vi "Get Revolutions.vi"(8 "error in (no error)":errorcluster, 11 "DriveMotors in":refnum<class "DriveMotors.lvclass">) -> (0 "error out":errorcluster, 2 "Revolutions":dbl, 3 "DriveMotors out":refnum<class "DriveMotors.lvclass">)   [LabVIEW 2013, in "DriveMotors.lvclass"]
uses:
  DriveMotors.lvclass
  DriveMotors.lvclass/DriveMotors.ctl
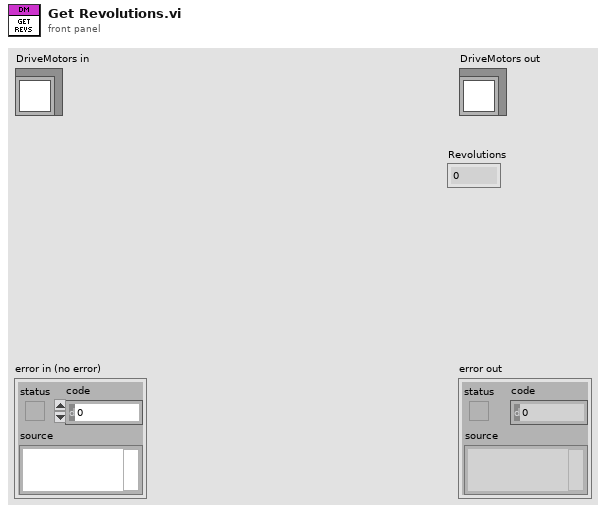
[diagram p1: front panel]
types:
  T1 = typedef "WPI_EncoderDevRef.ctl" = cluster{"DevStatus":errorcluster, "EncoderIndex":T2, "CounterIndex":T3, "DistancePerCount":dbl, "Decoding Type":T4}
  T2 = typedef "FPGA_EncoderIdx.ctl" = enum8{"Enc 0", "Enc 1", "Enc 2", "Enc 3", "Invalid"}
  T3 = typedef "FPGA_CounterCtrSystemIndex.ctl" = enum8{"Ctr 0", "Ctr 1", "Ctr 2", "Ctr 3", "Ctr 4", "Ctr 5", "Ctr 6", "Ctr 7", "Invalid"}
  T4 = typedef "WPI_EncoderType.ctl" = enum16{"1x", "2x", "4x"}
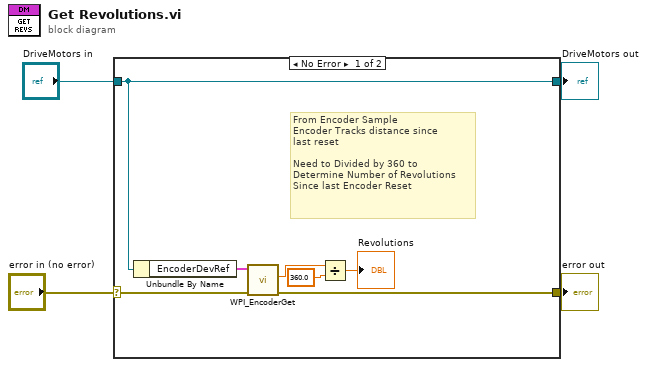
[diagram p0: block diagram]
diagram:
  n1 = case shown="No Error" "error in (no error)" {
    selector: "error in (no error)" -> [w6 w13]
    tunnel: [w5 w13] -> w3
    tunnel: [w11 w12] -> w1
    tunnel: "DriveMotors in" -> [w11 w12]
    frame No Error {
      # "From Encoder Sample\nEncoder Tracks distance since \nlast reset\n\nNeed to Divided by 360 to \nDetermine Number of Revolutions\nSince last Encoder Reset"
      n2 = Unbundle By Name(w11) -> ("EncoderDevRef"=w10:T1)
      n3 = call <vilib>:"WPI_EncoderGet.vi"("error in (no error)"=w6, "EncoderDevRef"=w10) -> ("error out"=w5:errorcluster, "Distance"=w8:dbl)  [unwired: 8 out]
      n4 = Divide(x=w8, y=360.0) -> (x/y=→"Revolutions":dbl)
    }
    frame Error {
    }
  }
  "error out" <- w3
  "DriveMotors out" <- w1
